vi "test_Multiple Periodic Command Message.vi"(8 "error in (no error)":errorcluster, 11 "TestCase in":refnum<class "Instrument Addon Common System Tests.lvclass">) -> (0 "error out":errorcluster, 3 "TestCase out":refnum<class "Instrument Addon Common System Tests.lvclass">)   [LabVIEW 2020, in "Instrument Addon Common System Tests.lvclass"]
uses:
  Instrument Addon Common System Tests.lvclass
  C:/Program Files (x86)/National Instruments/LabVIEW 2020/vi.lib/NI/VeriStand Custom Device Testing Tools/VeriStandTestCase/VeriStandTestCase.lvclass
  4b26bf46-6d54-4276-a8e8-45773f49de4b.vi
  <vilib>/addons/_JKI Toolkits/VI Tester/TestCase.llb/TestCase.lvclass
  C:/Program Files (x86)/National Instruments/LabVIEW 2020/vi.lib/addons/_JKI Toolkits/VI Tester/TestCase.llb/TestCase.lvclass
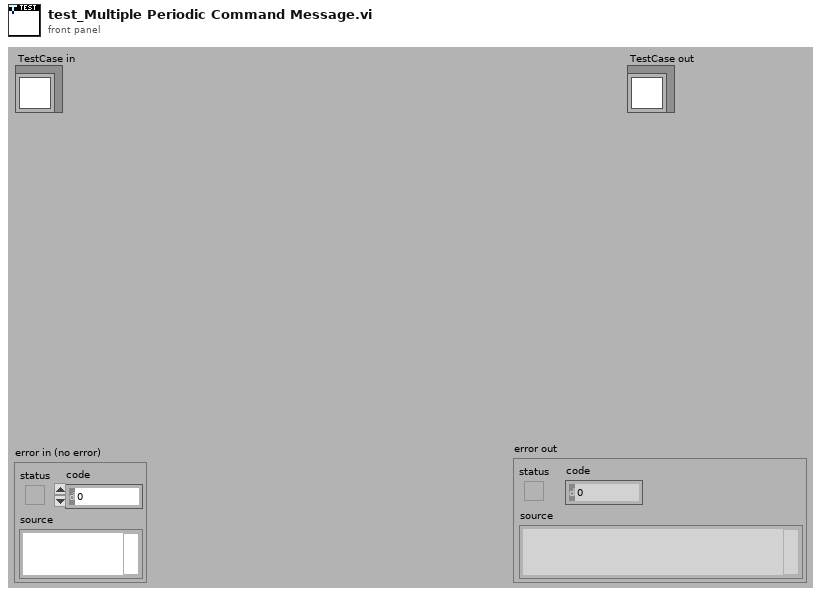
[diagram p1: front panel]
types:
  T1 = typedef "NI_VS Workspace ExecutionAPI.lvlib/WorkspaceAPI.ctl" = refnum<k24>
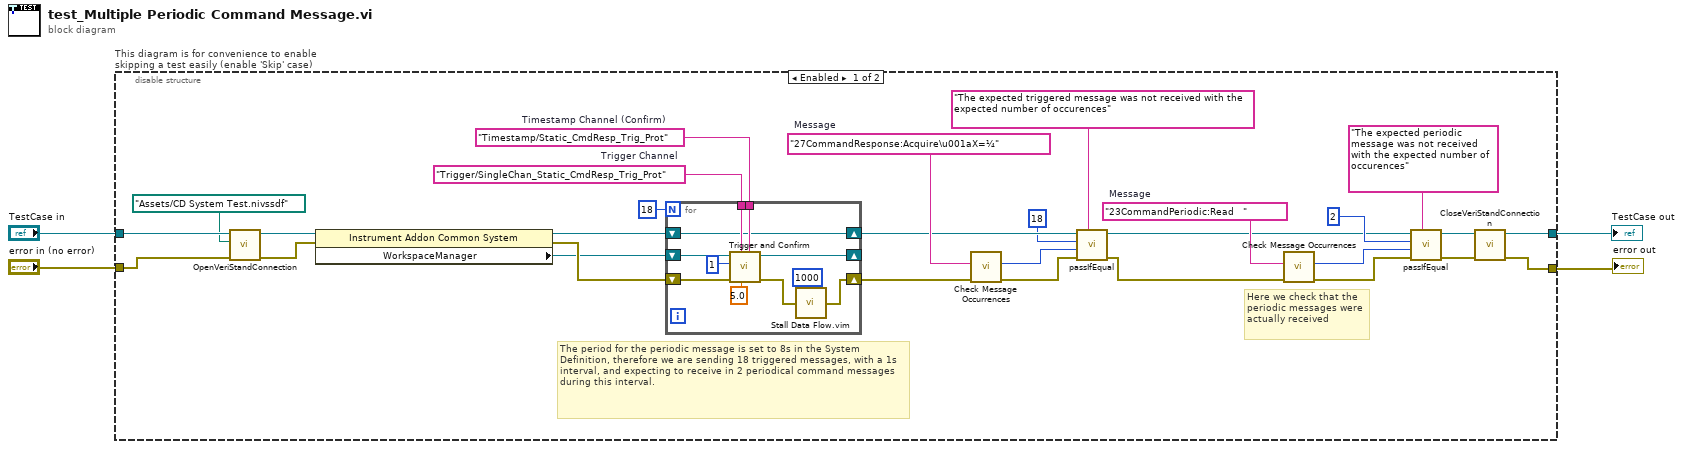
[diagram p0: block diagram]
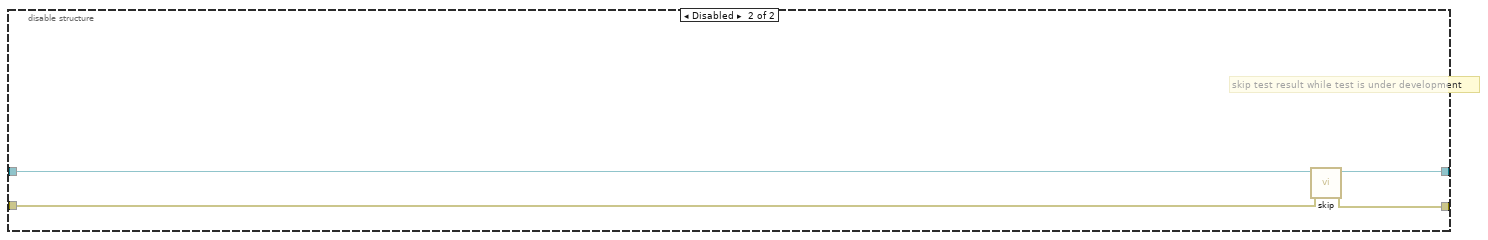
[diagram p2: hidden frame]
diagram:
  n1 = disable-structure "This diagram is for convenience to enable skipping a test easily (enable 'Skip' case)" shown="Enabled" {
    disable-tunnel: "TestCase in" -> [w31 w48]
    disable-tunnel: [w32 w46] -> w2
    disable-tunnel: [w33 w47] -> w1
    disable-tunnel: "error in (no error)" -> [w29 w45]
    frame Enabled {
      w12 = "27CommandResponse:Acquire\u001aX=¼"  # Message
      w20 = "Timestamp/Static_CmdResp_Trig_Prot"  # Timestamp Channel (Confirm)
      w19 = "Trigger/SingleChan_Static_CmdResp_Trig_Prot"  # Trigger Channel
      w21 = "23CommandPeriodic:Read   "  # Message
      # "The period for the periodic message is set to 8s in the System Definition, therefore we are sending 18 triggered messages, with a 1s interval, and expecting to receive in 2 periodical command messages during this interval."
      # "Here we check that the periodic messages were actually received"
      n2 = call-dynamic "OpenVeriStandConnection.vi"("error in (no error)"=w29, "System Definition File"=path "Assets/CD System Test.nivssdf", "VeriStand Test Case in"=w31) -> ("error out"=w28:errorcluster, "VeriStand Test Case out"=w30:refnum<class "Instrument Addon Common System Tests.lvclass">)  [unwired: 6 in, 1 out]
      n3 = property class="Instrument Addon Common System "(reference=w30, error in=w28) -> (reference out=w15:refnum<class "Instrument Addon Common System Tests.lvclass">, error out=w18:errorcluster, "WorkspaceManager"=w17:T1)
      n4 = for {
        N: 18 -> [_]
        tunnel: w20 -> [w44]
        tunnel: w19 -> [w43]
        shift-right: [w36] -> _
        shift-left: w17 -> [w40]
        shift-right: [w35] -> w13
        shift-left: w18 -> [w41]
        shift-right: [w34] -> w8
        shift-left: w15 -> [w34]
        n5 = call "Trigger and Confirm.vi"("Timestamp Channel (Confirm)"=w44, "Timeout (s)"=5.0, "Trigger Channel"=w43, "error in (no error)"=w41, "Number of Triggers"=1, "WorkspaceManager in"=w40) -> ("error out"=w39:errorcluster, "WorkspaceManager out"=w36:T1)  [unwired: 4 in]
        n6 = call "Stall Data Flow.vim"("value in"=w39, "milliseconds to wait"=u32 1000) -> ("value out"=w35:errorcluster)  [unwired: 1 out]
      }
      n7 = call "Check Message Occurrences.vi"("error in (no error)"=w13, "Message"=w12) -> ("error IO"=w11:errorcluster, "Occurences"=w10:i32)  [unwired: 8 in]
      n8 = call-dynamic "passIfEqual.vi"("custom report message (\"\")"="The expected triggered message was not received with the expected number of occurences" ("custom report message (\"\")"), "error in (no error)"=w11, "y"=w10, "x"=18 ("Occurences"), "TestCase in"=w8) -> ("error out"=w9:errorcluster, "TestCase out"=w7:refnum<class "Instrument Addon Common System Tests.lvclass">)  [unwired: 5 in]
      n9 = call "Check Message Occurrences.vi"("error in (no error)"=w9, "Message"=w21) -> ("error IO"=w26:errorcluster, "Occurences"=w23:i32)  [unwired: 8 in]
      n10 = call-dynamic "passIfEqual.vi"("custom report message (\"\")"="The expected periodic message was not received with the expected number of occurences" ("custom report message (\"\")"), "error in (no error)"=w26, "y"=w23, "x"=2, "TestCase in"=w7) -> ("error out"=w25:errorcluster, "TestCase out"=w14:refnum<class "Instrument Addon Common System Tests.lvclass">)  [unwired: 5 in]
      n11 = call-dynamic "CloseVeriStandConnection.vi"("error in (no error)"=w25, "VeriStand Test Case in"=w14) -> ("error out"=w33:errorcluster, "VeriStand Test Case out"=w32:refnum<class "Instrument Addon Common System Tests.lvclass">)  [unwired: 8 in]
    }
    frame Disabled {
      # "skip test result while test is under development"
      n12 = call <vilib>:"skip.vi"("error in (no error)"=w45, "TestCase in"=w48) -> ("error out"=w47:errorcluster, "TestCase out"=w46:refnum<class "Instrument Addon Common System Tests.lvclass">)  [unwired: 8 in]
    }
  }
  "error out" <- w1
  "TestCase out" <- w2
